vi "test Resource conflicts.vi"() -> ()   [LabVIEW 2016]
uses:
  CTL/Axis Data.ctl
  CTL/Motion IO.ctl
  CTL/Digital Lines (Read).ctl
  CTL/Status.ctl
  CTL/Encoder.ctl
  CTL/Position.ctl
  <vilib>/Motion/PropertyNodes/nimc.createStraightLineMoveInstance.axis.vi
  <vilib>/Motion/PropertyNodes/nimc.destroyInterfaceInstance.vi
  <resource>/objmgr/nimcca.rc
  SMD-7615.lvlib
  <resource>/objmgr/nimotion.rc
panel:
  in  "Position":dbl
  in  "Move":bool
  out "Axis Data":T1
  out "err out axis ref loop":errorcluster
  in  "Axis":refnum<k21>="niss:\\\\192.168.1.10"
  out "err out line ref loop":errorcluster
  in  "stop":bool
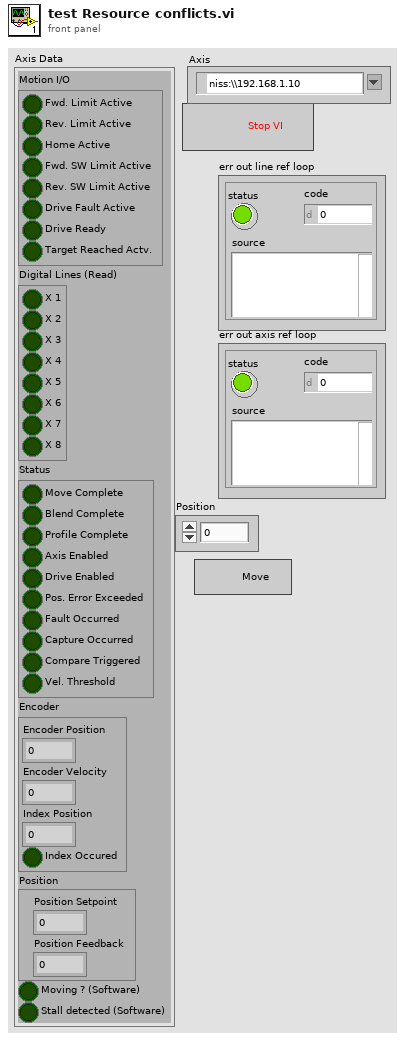
[diagram p1: front panel]
types:
  T1 = typedef "SMD-7615.lvlib/Axis Data.ctl" = cluster{"Motion I/O":T2, "Digital Lines (Read)":T3, "Status":T4, "Encoder":T5, "Position":T6, "Moving ? (Software)":bool, "Stall detected (Software)":bool}
  T2 = typedef "SMD-7615.lvlib/Motion IO.ctl" = cluster{"Fwd. Limit Active":bool, "Rev. Limit Active":bool, "Home Active":bool, "Fwd. SW Limit Active":bool, "Rev. SW Limit Active":bool, "Drive Fault Active":bool, "Drive Ready":bool, "Target Reached Actv.":bool}
  T3 = typedef "SMD-7615.lvlib/Digital Lines (Read).ctl" = cluster{"X 1":bool, "X 2":bool, "X 3":bool, "X 4":bool, "X 5":bool, "X 6":bool, "X 7":bool, "X 8":bool}
  T4 = typedef "SMD-7615.lvlib/Status.ctl" = cluster{"Move Complete":bool, "Blend Complete":bool, "Profile Complete":bool, "Axis Enabled":bool, "Drive Enabled":bool, "Pos. Error Exceeded":bool, "Fault Occurred":bool, "Capture Occurred":bool, "Compare Triggered":bool, "Vel. Threshold":bool}
  T5 = typedef "SMD-7615.lvlib/Encoder.ctl" = cluster{"Encoder Position":dbl, "Encoder Velocity":dbl, "Index Position":dbl, "Index Occured":bool}
  T6 = typedef "SMD-7615.lvlib/Position.ctl" = cluster{"Position Setpoint":dbl, "Position Feedback":dbl}
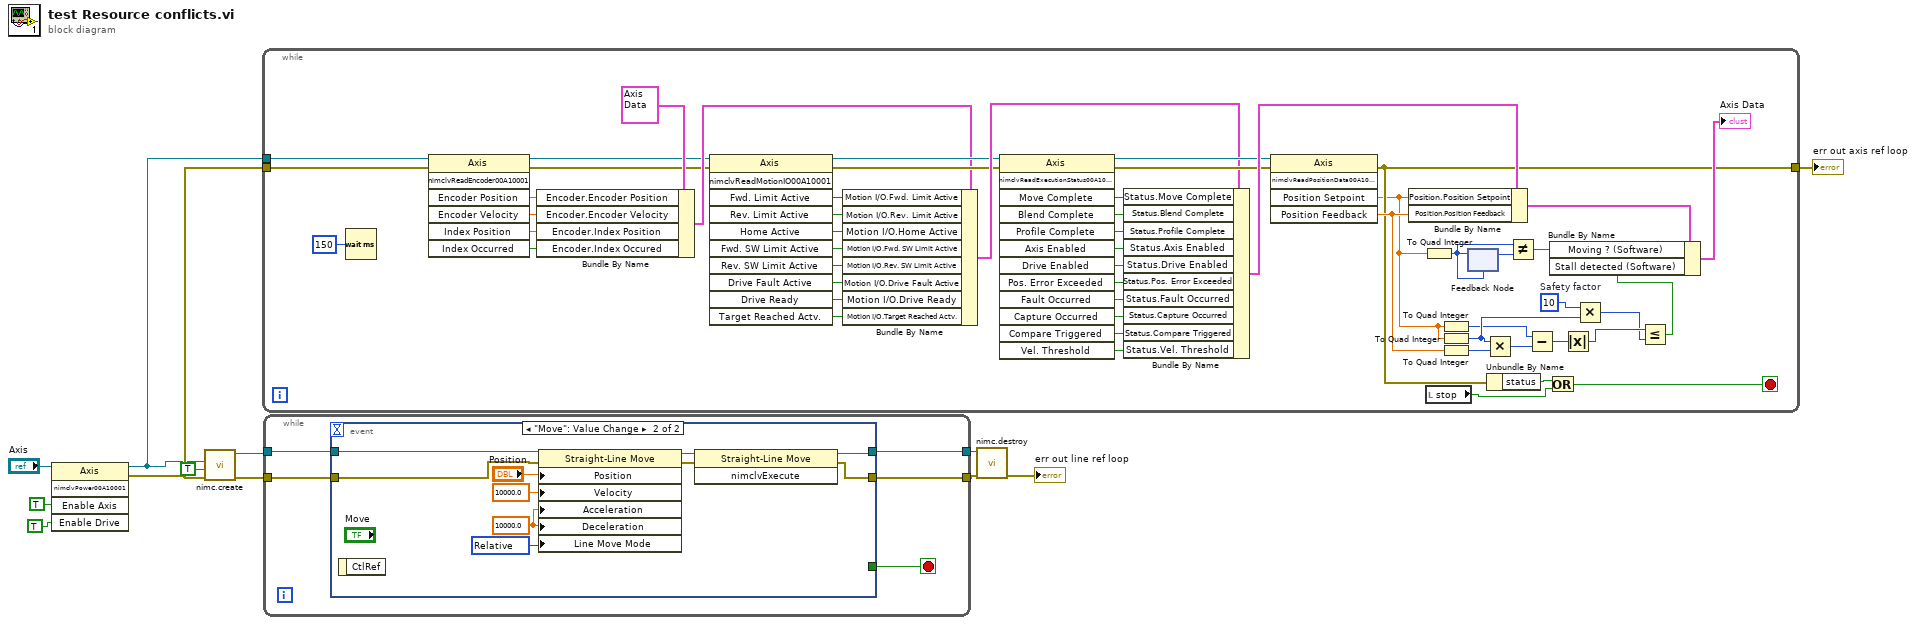
[diagram p0: block diagram]
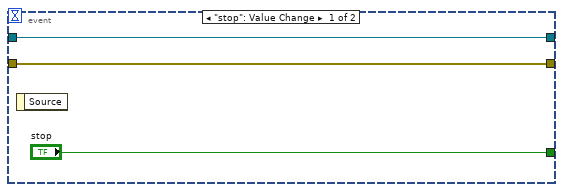
[diagram p2: hidden frame]
diagram:
  n1 = invoke class="Axis" method="nimclvPower00A10001"(reference="Axis", "Enable Axis"=TRUE, "Enable Drive"=TRUE ("Enable")) -> (reference out=w7:refnum<k21>, error out=w8:errorcluster)  [unwired: 2 in, 3 out]
  n2 = call-poly <vilib>:"nimc.create.vi"("error in"=w8, "async?"=TRUE, "axis"=w7) -> ("error out"=w11:errorcluster, "line"=w12:refnum<k20>)  [unwired: 6 in, 1 out]
  n3 = while {
    tunnel: w8 -> [w15]
    tunnel: w7 -> [w16]
    tunnel: [w19] -> w2
    stop <- w17 stop-if-true
    w62 = i64 10  # Safety factor
    n4 = Wait (ms)(milliseconds to wait=u32 150) -> ()  [unwired: 1 out]
    n5 = invoke class="Axis" method="nimclvReadEncoder00A10001"(reference=w16, error in=w15) -> (reference out=w22:refnum<k21>, error out=w21:errorcluster, "Encoder Position"=w23:dbl, "Encoder Velocity"=w24:dbl, "Index Position"=w25:dbl, "Index Occurred"=w26:bool)  [unwired: 5 in, 1 out]
    n6 = Bundle By Name(cluster=T1 {"Motion I/O"={"Fwd. Limit Active"=FALSE, "Rev. Limit Active"=FALSE, "Home Active"=FALSE, "Fwd. SW Limit Active"=FALSE, "Rev. SW Limit Active"=FALSE, "Drive Fault Active"=FALSE, "Drive Ready"=FALSE, "Target Reached Actv."=FALSE}, "Digital Lines (Read)"={"X 1"=FALSE, "X 2"=FALSE, "X 3"=FALSE, "X 4"=FALSE, "X 5"=FALSE, "X 6"=FALSE, "X 7"=FALSE, "X 8"=FALSE}, "Status"={"Move Complete"=FALSE, "Blend Complete"=FALSE, "Profile Complete"=FALSE, "Axis Enabled"=FALSE, "Drive Enabled"=FALSE, "Pos. Error Exceeded"=FALSE, "Fault Occurred"=FALSE, "Capture Occurred"=FALSE, "Compare Triggered"=FALSE, "Vel. Threshold"=FALSE}, "Encoder"={"Encoder Position"=0.0, "Encoder Velocity"=0.0, "Index Position"=0.0, "Index Occured"=FALSE}, "Position"={"Position Setpoint"=0.0, "Position Feedback"=0.0}, "Moving ? (Software)"=FALSE, "Stall detected (Software)"=FALSE} ("Axis Data"), "Encoder.Encoder Position"=w23, "Encoder.Encoder Velocity"=w24, "Encoder.Index Position"=w25, "Encoder.Index Occured"=w26) -> (w27:T1)
    n7 = invoke class="Axis" method="nimclvReadMotionIO00A10001"(reference=w22, error in=w21) -> (reference out=w36:refnum<k21>, error out=w37:errorcluster, "Fwd. Limit Active"=w28:bool, "Rev. Limit Active"=w29:bool, "Home Active"=w30:bool, "Fwd. SW Limit Active"=w31:bool, "Rev. SW Limit Active"=w32:bool, "Drive Fault Active"=w33:bool, "Drive Ready"=w34:bool, "Target Reached Actv."=w35:bool)  [unwired: 9 in, 1 out]
    n8 = Bundle By Name(cluster=w27, "Motion I/O.Fwd. Limit Active"=w28, "Motion I/O.Rev. Limit Active"=w29, "Motion I/O.Home Active"=w30, "Motion I/O.Fwd. SW Limit Active"=w31, "Motion I/O.Rev. SW Limit Active"=w32, "Motion I/O.Drive Fault Active"=w33, "Motion I/O.Drive Ready"=w34, "Motion I/O.Target Reached Actv."=w35) -> (w38:T1)
    n9 = invoke class="Axis" method="nimclvReadExecutionStatus00A10001"(reference=w36, error in=w37) -> (reference out=w50:refnum<k21>, error out=w49:errorcluster, "Move Complete"=w48:bool, "Blend Complete"=w47:bool, "Profile Complete"=w46:bool, "Axis Enabled"=w45:bool, "Drive Enabled"=w44:bool, "Pos. Error Exceeded"=w43:bool, "Fault Occurred"=w42:bool, "Capture Occurred"=w41:bool, "Compare Triggered"=w40:bool, "Vel. Threshold"=w39:bool)  [unwired: 11 in, 1 out]
    n10 = Bundle By Name(cluster=w38, "Status.Move Complete"=w48, "Status.Blend Complete"=w47, "Status.Profile Complete"=w46, "Status.Axis Enabled"=w45, "Status.Drive Enabled"=w44, "Status.Pos. Error Exceeded"=w43, "Status.Fault Occurred"=w42, "Status.Capture Occurred"=w41, "Status.Compare Triggered"=w40, "Status.Vel. Threshold"=w39) -> (w51:T1)
    n11 = invoke class="Axis" method="nimclvReadPositionData00A10001"(reference=w50, error in=w49) -> (error out=w19:errorcluster, "Position Setpoint"=w14:dbl, "Position Feedback"=w56:dbl)  [unwired: 3 in, 2 out]
    n12 = Bundle By Name(cluster=w51, "Position.Position Setpoint"=w14, "Position.Position Feedback"=w56) -> (w52:T1)
    n13 = To Quad Integer(1:w14) -> (0:w53:i64)
    n14 = local read "stop"() -> (w13:bool)
    n15 = To Quad Integer(1:w14) -> (0:w60:i64)
    n16 = To Quad Integer(1:w14) -> (0:w63:i64)
    n17 = To Quad Integer(1:w56) -> (0:w57:i64)
    n18 = feedback #1(w53) -> (w55:i64)
    n19 = feedback-in #1(w53) -> ()
    n20 = Multiply(x=w63, y=w57) -> (x*y=w58:i64)
    n21 = Unbundle By Name(w19) -> ("status"=w18:bool)
    n22 = Not Equal?(x=w53, y=w55) -> (x != y?=w54:bool)
    n23 = Subtract(x=w60, y=w58) -> (x-y=w59:i64)
    n24 = Or(x=w18, y=w13) -> (x .or. y?=w17:bool)
    n25 = Absolute Value(x=w59) -> (abs(x)=w65:i64)
    n26 = Multiply(x=w62, y=w63) -> (x*y=w64:i64)
    n27 = Less Or Equal?(x=w65, y=w64) -> (x <= y?=w61:bool)
    n28 = Bundle By Name(cluster=w52, "Moving ? (Software)"=w54, "Stall detected (Software)"=w61) -> (→"Axis Data":T1)
  }
  "err out axis ref loop" <- w2
  n29 = while {
    tunnel: w12 -> [w71]
    tunnel: w11 -> [w69]
    tunnel: [w72] -> w4
    tunnel: [w70] -> w3
    stop <- w68 stop-if-true
    n30 = event shown="[1] \"Move\": Value Change" {
      selector: _ -> [_ _]
      dyn-events: _ -> [_ _]
      timeout: _ -> [_ _]
      tunnel: [w75 w83] -> w72
      tunnel: w71 -> [w75 w76]
      tunnel: [w74 w82] -> w70
      tunnel: w69 -> [w74 w77]
      tunnel: ["stop" _] -> w68
      event "stop": Value Change {
        n31 = event-data() -> ()  [unwired: 1 in, 1 out]
      }
      event "Move": Value Change {
        w80 = 10000.0 ("Deceleration")
        w81 = 10551344 items=["Relative"=10551344, "Absolute"=10551337, "Relative To Capture"=10551345, "Velocity"=10551346, "Polyline"=11600101] ("Line Move Mode")
        n32 = event-data() -> ()  [unwired: 1 in, 1 out]
        n33 = property class="Straight-Line Move"(reference=w76, error in=w77, "Position"="Position", "Velocity"=10000.0, "Acceleration"=w80, "Deceleration"=w80, "Line Move Mode"=w81) -> (reference out=w85:refnum<k20>, error out=w84:errorcluster)
        n34 = invoke class="Straight-Line Move" method="nimclvExecute"(reference=w85, error in=w84) -> (reference out=w83:refnum<k20>, error out=w82:errorcluster)  [unwired: 1 in, 1 out]
      }
    }
  }
  n35 = call-poly <vilib>:"nimc.destroy.vi"("error in"=w3, "motion handle"=w4) -> ("error out"=→"err out line ref loop":errorcluster)  [unwired: 9 in]
